vi "7.1.vi"() -> ()   [LabVIEW 2017]
uses:
  <vilib>/Analysis/NI_AALBase.lvlib
panel:
  out "min value":i32
  out "max value":i32
  out "sum":i32
  out "array":i32[](array[numeric])
  in  "String":string
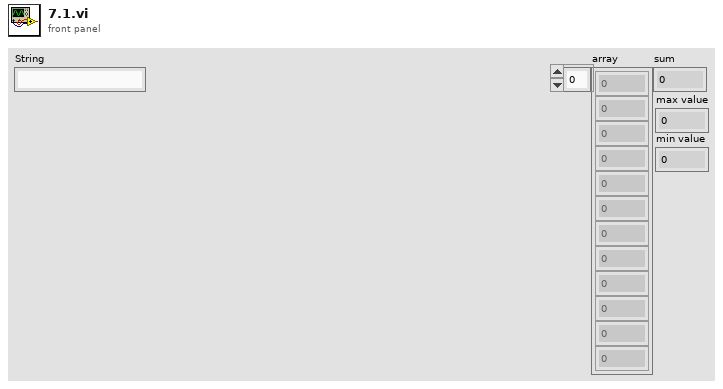
[diagram p1: front panel]
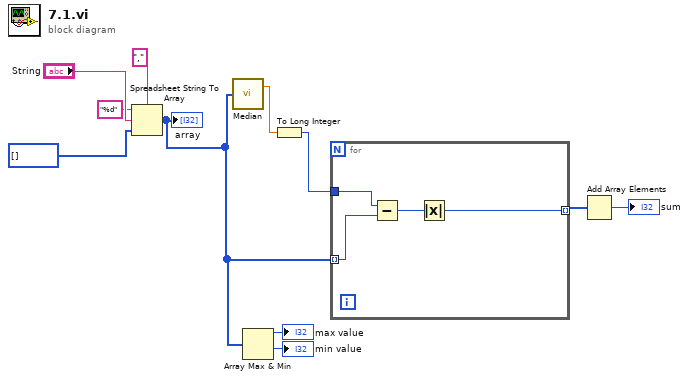
[diagram p0: block diagram]
diagram:
  n1 = Spreadsheet String To Array(delimiter (Tab)=",", format string="%d", spreadsheet string="String", array type (2D Dbl)=i32[] []) -> (array=w3:i32[])
  "array" <- w3
  n2 = call <vilib>:"Median.vi"("X"=w3) -> ("median"=w7:dbl)  [unwired: 1 out]
  n3 = Array Max & Min(array=w3) -> (max value=→"max value":i32, min value=→"min value":i32)  [unwired: 2 out]
  n4 = To Long Integer(number=w7) -> (32bit integer=w6:i32)
  n5 = for {
    tunnel: w6 -> [w15]
    tunnel: w3 -> [w14] mode=indexing
    tunnel: [w12] -> w5 mode=indexing
    n6 = Subtract(x=w15, y=w14) -> (x-y=w13:i32)
    n7 = Absolute Value(x=w13) -> (abs(x)=w12:i32)
  }
  n8 = Add Array Elements(numeric array=w5) -> (sum=→"sum":i32)
